vi "DW Test Change Info.vi"(10 "evl":u32(ring) items=["good", "middle", "bad"], 11 "member":T1) -> (1 "name":string, 2 "evl out":u32(ring) items=["good", "middle", "bad"], 3 "member out":T1)   [LabVIEW 2020, in "ImportSharedLibraryExample.lvlib"]
doc: "void DWTest_Change_Info(MemberInfo* member, evaluation* evl );"
uses:
  ImportSharedLibraryExample.lvlib
  <vilib>/Utility/importsl/GetValueByPointer/GetValueByPointer.xnode
  ImportSharedLibraryExample.dll
  <resource>/lvimptsl.dll
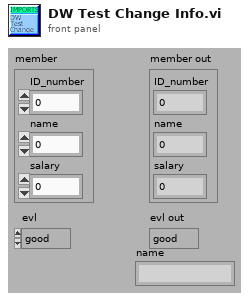
[diagram p1: front panel]
types:
  T1 = cluster{"ID_number":i32, "name":u32, "salary":i32}
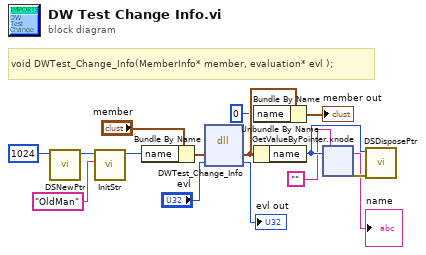
[diagram p0: block diagram]
diagram:
  # "void DWTest_Change_Info(MemberInfo* member, evaluation* evl );"
  n1 = call <vilib>:"DSNewPtr.vi"("Size"=u64 1024) -> ("Pointer"=w13:u64)  [unwired: 1 in, 9 out]
  n2 = call <vilib>:"InitStr.vi"("ConstCStr"="OldMan", "Pointer"=w13) -> ("CStrP"=w11:u64)  [unwired: 1 in, 8 out]
  n3 = Bundle By Name(cluster="member", "name"=w11) -> (w10:T1)
  n4 = dll-call lib="e:/builds/penguin/labview/branches/2020/dev/dist/examples/dll/ImportSharedLibraryExample/ImportSharedLibraryExample.*" fn="DWTest_Change_Info"("member"=w10, "evl"="evl") -> ("member"=w5:T1, "evl"=→"evl out":u32)  [unwired: 3 in, 3 out]
  n5 = Bundle By Name(cluster=w5, "name"=u32 0) -> (→"member out":T1)
  n6 = Unbundle By Name(w5) -> ("name"=w8:u32)
  n7 = xnode "GetValueByPointer.xnode"("Pointer"=w8, "InputType"="") -> ("Output"=→"name":string, "ErrorOut"=w9:errorcluster)  [unwired: 2 in]
  n8 = call <vilib>:"DSDisposePtr.vi"("error in (no error)"=w9, "Pointer"=w8) -> ()  [unwired: 10 out]
